vi "CSM - Read File Logger Configuration from INI String.vi"   [LabVIEW 2017, in "INI-Static-Variable-Support.lvlib"]
doc: "Reads log recording configuration from the configuration. This configuration is primarily used with the following VI:\n\n- `addons\\Logger\\CSM - Start File Logger.vi`"
uses:
  INI-Static-Variable-Support.lvlib
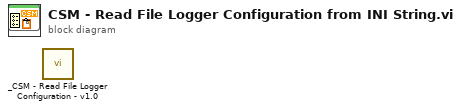
[diagram p0: block diagram]
diagram:
  n1 = call "_CSM - Read File Logger Configuration - v1.0.vi"() -> ()  [unwired: 8 in, 2 out]
